vi "Write AE.vi"(8 "error in (no error)":errorcluster, 10 "AE":refnum<class "AE.lvclass">, 11 "CS++AEUpdate Msg in":refnum<class "CS++AEUpdate Msg.lvclass">) -> (0 "error out":errorcluster, 3 "CS++AEUpdate Msg out":refnum<class "CS++AEUpdate Msg.lvclass">)   [LabVIEW 2014, in "CS++PVMonitor.lvlib" / "CS++AEUpdate Msg.lvclass"]
doc: "Write PV."
uses:
  CS++AEUpdate Msg.lvclass
  Classes/CS++ProcessVariables/AlarmEvent/AE.lvclass
  CS++AEUpdate Msg.lvclass/CS++AEUpdate Msg.ctl
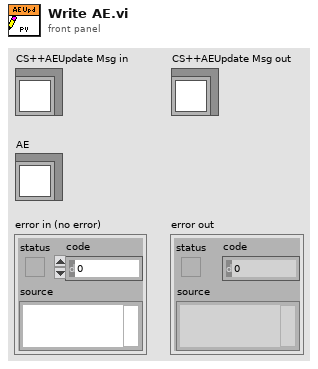
[diagram p1: front panel]
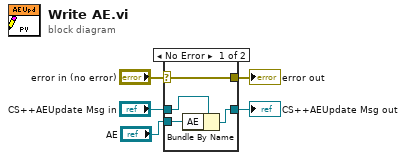
[diagram p0: block diagram]
diagram:
  n1 = case shown="No Error" "error in (no error)" {
    selector: "error in (no error)" -> [w9 w10]
    tunnel: [w9 w10] -> w4
    tunnel: [w7 w11] -> w2
    tunnel: "CS++AEUpdate Msg in" -> [w8 w11]
    tunnel: "AE" -> [w6 _]
    frame No Error {
      n2 = Bundle By Name(cluster=w8, "AE"=w6) -> (w7:refnum<class "CS++AEUpdate Msg.lvclass">)
    }
    frame Error {
    }
  }
  "error out" <- w4
  "CS++AEUpdate Msg out" <- w2
